vi "ControlFifoImage.vi"(7 "CloseReferences(F)":bool, 8 "ErrorIn":errorcluster, 11 "Job-Command":string) -> (0 "ErrorOut":errorcluster, 1 "ResultCtlRef":refnum<vi>, 2 "UserInputRef":refnum<vi>, 3 "ButtonRefs":T1, 5 "IntensityImageRef":refnum<vi>)   [LabVIEW 2023]
doc: "This VI searches and provides refnums to controls/indicators in FifoImage. Use this VI to remotely control FifoImage.exe from your own VI.\nAn example use scenario is shown in RemoteControlFifoImage.vi\nFifoImage.exe opens Port 3366\n\ninfo@becker-hickl.com"
panel:
  out "JobCtlRef":refnum<vi>
  out "vi ref":refnum<vi>
  out "application ref":refnum<vi>
  # "3580 is in LabView USE"
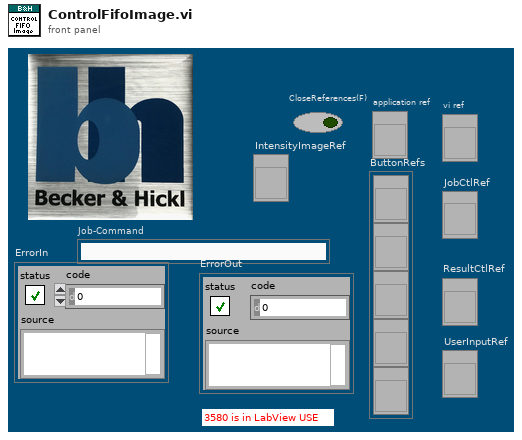
[diagram p1: front panel]
types:
  T1 = cluster{refnum<vi>, refnum<vi>, refnum<vi>, refnum<vi>, refnum<vi>}
  T2 = cluster{"IsError(T)":bool, "code":i32, "ResultIn":string}
  T3 = cluster{refnum<k0>, refnum<k0>, refnum<k0>, refnum<k0>, refnum<k0>}
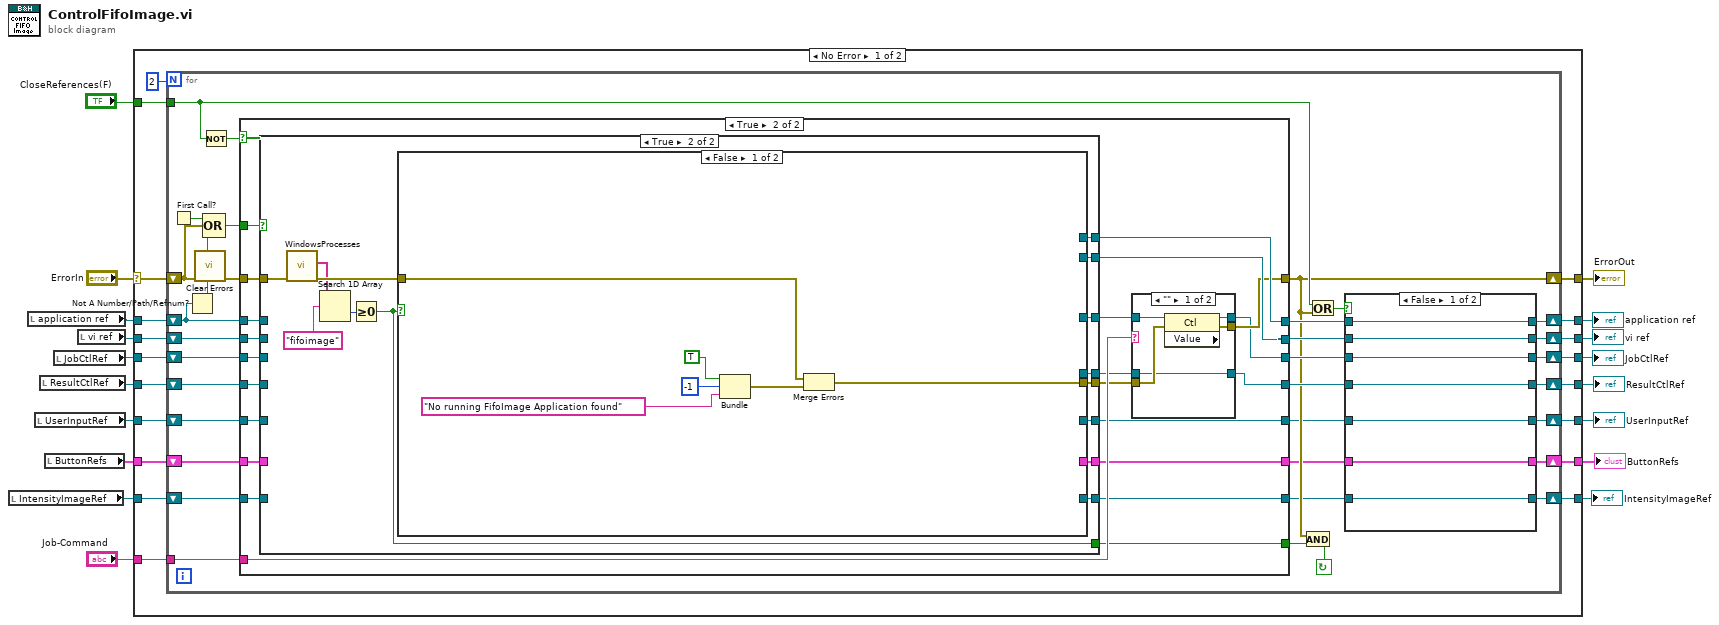
[diagram p0: block diagram]
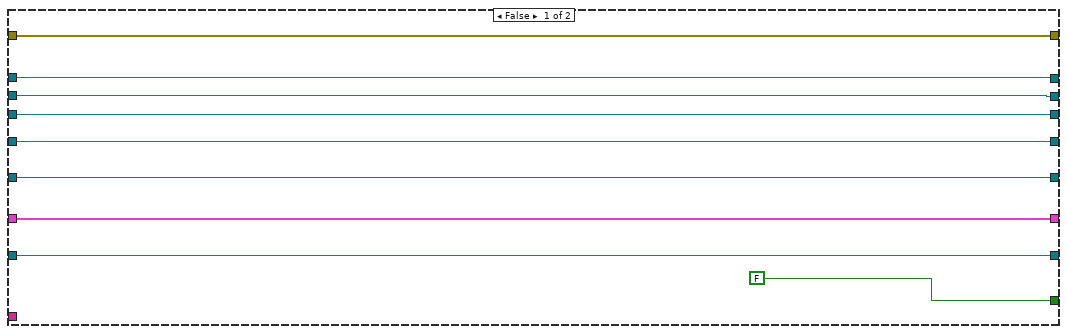
[diagram p2: hidden frame]
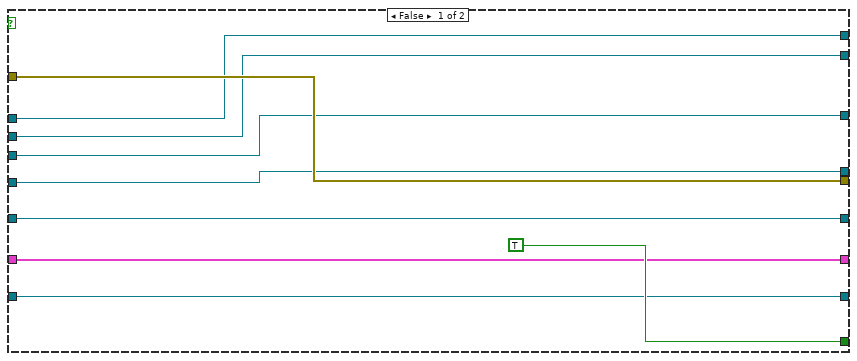
[diagram p3: hidden frame]
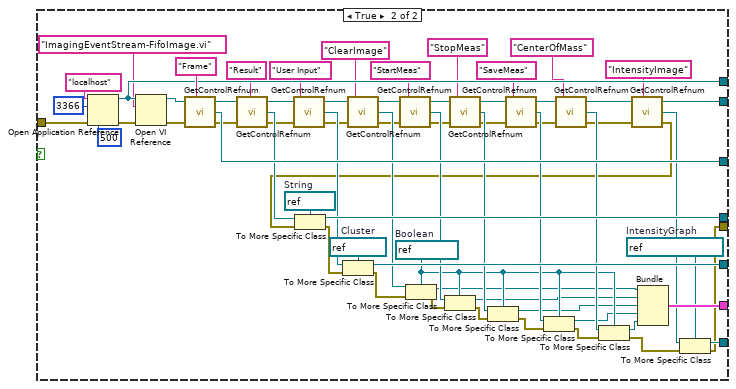
[diagram p4: hidden frame]
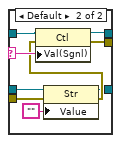
[diagram p5: hidden frame]
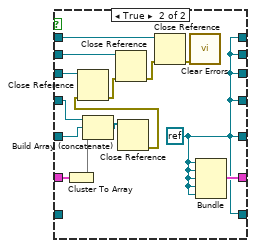
[diagram p6: hidden frame]
diagram:
  n1 = local read "IntensityImageRef"() -> (w1:refnum<vi>)
  n2 = local read "application ref"() -> (w7:refnum<vi>)
  n3 = local read "UserInputRef"() -> (w6:refnum<vi>)
  n4 = local read "ResultCtlRef"() -> (w14:refnum<vi>)
  n5 = local read "ButtonRefs"() -> (w3:T1)
  n6 = local read "JobCtlRef"() -> (w11:refnum<vi>)
  n7 = local read "vi ref"() -> (w9:refnum<vi>)
  n8 = case shown="No Error" "ErrorIn" {
    selector: "ErrorIn" -> [w34 w239]
    tunnel: "Job-Command" -> [w37 _]
    tunnel: [w36 w239] -> w17
    tunnel: "CloseReferences(F)" -> [w35 _]
    tunnel: w14 -> [w32 w238]
    tunnel: [w31 w238] -> w13
    tunnel: [w30 w237] -> w12
    tunnel: w11 -> [w29 w237]
    tunnel: [w28 w236] -> w10
    tunnel: w9 -> [w27 w236]
    tunnel: [w26 w235] -> w8
    tunnel: w7 -> [w25 w235]
    tunnel: [w24 w234] -> w5
    tunnel: w6 -> [w23 w234]
    tunnel: [w22 w233] -> w4
    tunnel: w3 -> [w21 w233]
    tunnel: [w20 w232] -> w2
    tunnel: w1 -> [w19 w232]
    frame No Error {
      n9 = for {
        N: 2 -> [_]
        tunnel: w37 -> [w70]
        shift-right: [w60] -> w26
        shift-left: w25 -> [w68]
        shift-right: [w59] -> w28
        shift-left: w27 -> [w67]
        shift-right: [w58] -> w30
        shift-left: w29 -> [w66]
        shift-right: [w53] -> w36
        shift-left: w34 -> [w57]
        tunnel: w35 -> [w61]
        shift-right: [w54] -> w31
        shift-left: w32 -> [w55]
        shift-right: [w45] -> w24
        shift-left: w23 -> [w44]
        shift-right: [w42] -> w22
        shift-left: w21 -> [w41]
        shift-right: [w39] -> w20
        shift-left: w19 -> [w38]
        stop <- w48 continue-if-true
        n10 = First Call?() -> (First Call?: T/F=w69:bool)
        n11 = Not A Number/Path/Refnum?(number/path/refnum=w68) -> (NaN/Path/Refnum?=w49:bool)
        n12 = call <vilib>:"Clear Errors.vi"("error in (no error)"=w57) -> ("error out"=w51:errorcluster)  [unwired: 1 in, 5 out]
        n13 = Not(x=w61) -> (.not. x?=w50:bool)
        n14 = Compound Arithmetic op=OR(w69, w57, w49) -> (w52:bool)
        n15 = case shown="True" w50 {
          tunnel: w51 -> [w79 w101]
          tunnel: w70 -> [_ w95]
          tunnel: [w79 w88] -> w53
          tunnel: w52 -> [_ w100]
          tunnel: w68 -> [w78 w99]
          tunnel: w67 -> [w77 w98]
          tunnel: w66 -> [w76 w97]
          tunnel: [w78 w92] -> w63
          tunnel: [w77 w93] -> w64
          tunnel: [w76 w86] -> w65
          tunnel: w55 -> [w75 w96]
          tunnel: [w75 w89] -> w56
          tunnel: [FALSE w94] -> w47
          tunnel: [w73 w85] -> w46
          tunnel: w44 -> [w73 w84]
          tunnel: [w72 w83] -> w43
          tunnel: w41 -> [w72 w82]
          tunnel: [w71 w81] -> w40
          tunnel: w38 -> [w71 w80]
          frame False {
          }
          frame True {
            n16 = case shown="True" w100 {
              tunnel: [w110 w120] -> w91
              tunnel: w101 -> [w110 w119]
              tunnel: w99 -> [w109 _]
              tunnel: w98 -> [w108 _]
              tunnel: w97 -> [w107 _]
              tunnel: [w109 w124] -> w92
              tunnel: [w108 w122] -> w93
              tunnel: [w107 w123] -> w87
              tunnel: w96 -> [w106 _]
              tunnel: [w106 w121] -> w90
              tunnel: [TRUE w117] -> w94
              tunnel: [w104 w113] -> w85
              tunnel: w84 -> [w104 _]
              tunnel: [w103 w112] -> w83
              tunnel: w82 -> [w103 _]
              tunnel: [w102 w111] -> w81
              tunnel: w80 -> [w102 _]
              frame False {
              }
              frame True {
                n17 = call "WindowsProcesses.vi"("error in (no error)"=w119) -> ("error out"=w118:errorcluster, "ProcessNames"=w115:string[])  [unwired: 9 out]
                n18 = Search 1D Array(1D array=w115, element="fifoimage") -> (index of element=w116:i32)  [unwired: 1 in]
                n19 = Greater Or Equal To 0?(x=w116) -> (x >= 0?=w117:bool)
                n20 = case shown="False" w117 {
                  tunnel: w118 -> [w125 w194]
                  tunnel: [_ w192] -> w124
                  tunnel: [_ w191] -> w123
                  tunnel: [_ w151] -> w122
                  tunnel: [_ w185] -> w121
                  tunnel: [w126 w132] -> w120
                  tunnel: [_ w175] -> w113
                  tunnel: [_ w153] -> w112
                  tunnel: [_ w148] -> w111
                  frame False {
                    n21 = Bundle("IsError(T)"=TRUE, "code"=-1, "ResultIn"="No running FifoImage Application found") -> (w129:T2)  [unwired: 1 out]
                    n22 = Merge Errors(w125, w129) -> (w126:errorcluster)
                  }
                  frame True {
                    w149 = refnum<vi> refnum  # IntensityGraph
                    w159 = refnum<vi> refnum  # Boolean
                    w177 = refnum<vi> refnum  # Cluster
                    w187 = refnum<vi> refnum  # String
                    n23 = Open Application Reference(8:w194, 9:500 ("timeout ms (60000)"), 10:u32 3366, 11:"localhost" ("machine name (\"\":  open local reference)")) -> (0:w183:errorcluster, 3:w192:refnum<vi>)
                    n24 = Open VI Reference(application reference (local)=w192, vi path="ImagingEventStream-FifoImage.vi" ("ControlLabelText"), error in (no error)=w183) -> (vi reference=w193:refnum<vi>, error out=w195:errorcluster)  [unwired: 3 out]
                    n25 = call "GetControlRefnum.vi"("ErrorIn"=w195, "ControlLabelText"="Frame", "VIRefnumIn"=w193) -> ("ErrorOut"=w190:errorcluster, "CtlRefnum"=w191:refnum<vi>, "VIRefnumThru"=w189:refnum<vi>)
                    n26 = call "GetControlRefnum.vi"("ErrorIn"=w190, "ControlLabelText"="Result", "VIRefnumIn"=w189) -> ("ErrorOut"=w141:errorcluster, "CtlRefnum"=w186:refnum<vi>, "VIRefnumThru"=w178:refnum<vi>)
                    n27 = call "GetControlRefnum.vi"("ErrorIn"=w141, "ControlLabelText"="User Input", "VIRefnumIn"=w178) -> ("ErrorOut"=w147:errorcluster, "CtlRefnum"=w176:refnum<vi>, "VIRefnumThru"=w169:refnum<vi>)
                    n28 = call "GetControlRefnum.vi"("ErrorIn"=w147, "ControlLabelText"="ClearImage", "VIRefnumIn"=w169) -> ("ErrorOut"=w146:errorcluster, "CtlRefnum"=w164:refnum<vi>, "VIRefnumThru"=w171:refnum<vi>)
                    n29 = call "GetControlRefnum.vi"("ErrorIn"=w146, "ControlLabelText"="StartMeas", "VIRefnumIn"=w171) -> ("ErrorOut"=w145:errorcluster, "CtlRefnum"=w163:refnum<vi>, "VIRefnumThru"=w174:refnum<vi>)
                    n30 = call "GetControlRefnum.vi"("ErrorIn"=w145, "ControlLabelText"="StopMeas", "VIRefnumIn"=w174) -> ("ErrorOut"=w144:errorcluster, "CtlRefnum"=w162:refnum<vi>, "VIRefnumThru"=w166:refnum<vi>)
                    n31 = call "GetControlRefnum.vi"("ErrorIn"=w144, "ControlLabelText"="SaveMeas", "VIRefnumIn"=w166) -> ("ErrorOut"=w143:errorcluster, "CtlRefnum"=w161:refnum<vi>, "VIRefnumThru"=w167:refnum<vi>)
                    n32 = call "GetControlRefnum.vi"("ErrorIn"=w143, "ControlLabelText"="CenterOfMass", "VIRefnumIn"=w167) -> ("ErrorOut"=w142:errorcluster, "CtlRefnum"=w160:refnum<vi>, "VIRefnumThru"=w152:refnum<vi>)
                    n33 = call "GetControlRefnum.vi"("ErrorIn"=w142, "ControlLabelText"="IntensityImage", "VIRefnumIn"=w152) -> ("ErrorOut"=w140:errorcluster, "CtlRefnum"=w150:refnum<vi>, "VIRefnumThru"=w151:refnum<vi>)
                    n34 = To More Specific Class(target class=w187, reference=w186, error in=w140) -> (specific class reference=w185:refnum<vi>, error out=w139:errorcluster)
                    n35 = To More Specific Class(target class=w177, reference=w176, error in=w139) -> (specific class reference=w175:refnum<vi>, error out=w138:errorcluster)
                    n36 = To More Specific Class(target class=w159, reference=w164, error in=w138) -> (specific class reference=w158:refnum<vi>, error out=w137:errorcluster)
                    n37 = To More Specific Class(target class=w159, reference=w163, error in=w137) -> (specific class reference=w157:refnum<vi>, error out=w136:errorcluster)
                    n38 = To More Specific Class(target class=w159, reference=w162, error in=w136) -> (specific class reference=w156:refnum<vi>, error out=w135:errorcluster)
                    n39 = To More Specific Class(target class=w159, reference=w161, error in=w135) -> (specific class reference=w155:refnum<vi>, error out=w134:errorcluster)
                    n40 = To More Specific Class(target class=w159, reference=w160, error in=w134) -> (specific class reference=w154:refnum<vi>, error out=w133:errorcluster)
                    n41 = Bundle(w158, w157, w156, w155, w154) -> (w153:T1)  [unwired: 1 in]
                    n42 = To More Specific Class(target class=w149, reference=w150, error in=w133) -> (specific class reference=w148:refnum<vi>, error out=w132:errorcluster)
                  }
                }
              }
            }
            n43 = case shown="\"\"" w95 {
              selector: w95 -> [_ w207]
              tunnel: w87 -> [w201 w210]
              tunnel: [w200 w209] -> w86
              tunnel: [w199 w208] -> w88
              tunnel: w91 -> [w198 w205]
              tunnel: w90 -> [w197 w203]
              tunnel: [w197 w202] -> w89
              frame "" {
                n44 = property class="Ctl" props=["Value"](reference=w201, error in=w198) -> (reference out=w200:refnum<vi>, error out=w199:errorcluster)  [unwired: 1 out]
              }
              frame Default {
                n45 = property class="Str"(reference=w203, error in=w205, "Value"="") -> (reference out=w202:refnum<vi>, error out=w204:errorcluster)
                n46 = property class="Ctl"(reference=w210, error in=w204, "Val(Sgnl)"=w207) -> (reference out=w209:refnum<vi>, error out=w208:errorcluster)
              }
            }
          }
        }
        n47 = And(x=w53, y=w47) -> (x .and. y?=w48:bool)
        n48 = Or(x=w61, y=w53) -> (x .or. y?=w62:bool)
        n49 = case shown="False" w62 {
          tunnel: w65 -> [w215 w226]
          tunnel: w64 -> [w216 w225]
          tunnel: w63 -> [w217 w224]
          tunnel: [w217 w218] -> w60
          tunnel: [w216 w218] -> w59
          tunnel: [w215 w218] -> w58
          tunnel: w56 -> [w214 w227]
          tunnel: [w214 w218] -> w54
          tunnel: w46 -> [w213 w222]
          tunnel: [w213 w218] -> w45
          tunnel: w43 -> [w212 w221]
          tunnel: [w212 w219] -> w42
          tunnel: [w211 w218] -> w39
          tunnel: w40 -> [w211 _]
          frame False {
          }
          frame True {
            w218 = refnum<k0> refnum
            n50 = Cluster To Array(cluster=w221) -> (array=w220:refnum<vi>[])
            n51 = Build Array (concatenate)(w227, w222, w220) -> (w223:refnum<vi>[])
            n52 = Close Reference(reference=w223) -> (error out=w228:errorcluster)  [unwired: 1 in]
            n53 = Close Reference(reference=w226, error in (no error)=w228) -> (error out=w229:errorcluster)
            n54 = Close Reference(reference=w225, error in (no error)=w229) -> (error out=w230:errorcluster)
            n55 = Close Reference(reference=w224, error in (no error)=w230) -> (error out=w231:errorcluster)
            n56 = call <vilib>:"Clear Errors.vi"("error in (no error)"=w231) -> ()  [unwired: 1 in, 6 out]
            n57 = Bundle(w218, w218, w218, w218, w218) -> (w219:T3)  [unwired: 1 in]
          }
        }
      }
    }
    frame Error {
    }
  }
  "ErrorOut" <- w17
  "ResultCtlRef" <- w13
  "JobCtlRef" <- w12
  "vi ref" <- w10
  "application ref" <- w8
  "UserInputRef" <- w5
  "ButtonRefs" <- w4
  "IntensityImageRef" <- w2
